vi "UDP Send and Receive (repeat on error) - I32.vi"(7 "timeout ms (100)":i32=100, 8 "error in (no error)":errorcluster, 9 "I32 Command & Param":T1, 10 "IP":string, 11 "connection ID in":refnum<k16>) -> (0 "error out":errorcluster, 2 "I32 Param out":i32, 3 "connection ID out":refnum<k16>)   [LabVIEW 2016, in "SMD-7615.lvlib" / "eSCL.lvlib"]
doc: "AC - Acceleration Rate\nSets or requests the acceleration rate used in point-to-point move commands in rev/sec/sec."
uses:
  eSCL.lvlib
  I32 Command and Param.ctl
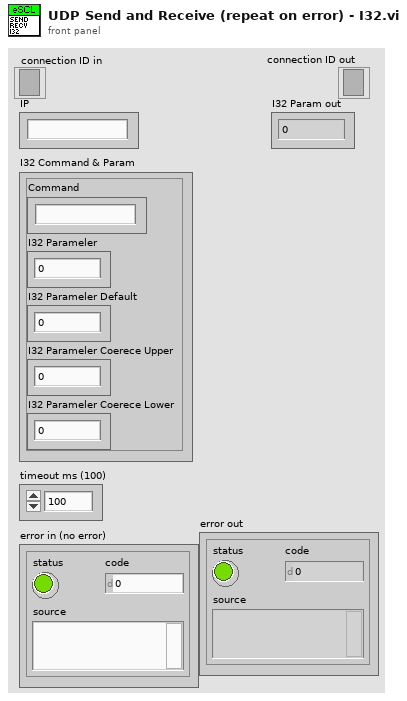
[diagram p1: front panel]
types:
  T1 = typedef "SMD-7615.lvlib/eSCL.lvlib/I32 Command and Param.ctl" = cluster{"Command":string, "I32 Parameler":i32, "I32 Parameler Default":i32, "I32 Parameler Coerece Upper":i32, "I32 Parameler Coerece Lower":i32}
  T2 = typedef "SMD-7615.lvlib/eSCL.lvlib/UDP Received Data.ctl" = cluster{"Received String":string, "eSCL Cmd":string, "Data":string}
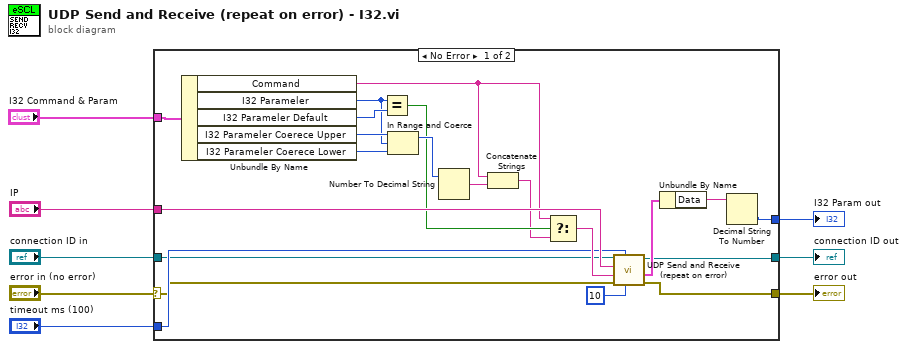
[diagram p0: block diagram]
diagram:
  n1 = case shown="No Error" "error in (no error)" {
    selector: "error in (no error)" -> [w11 w30]
    tunnel: "connection ID in" -> [w10 w31]
    tunnel: [w27 w31] -> w6
    tunnel: [w26 w30] -> w5
    tunnel: "IP" -> [w29 _]
    tunnel: "timeout ms (100)" -> [w12 _]
    tunnel: [w18 _] -> w2
    tunnel: "I32 Command & Param" -> [w25 _]
    frame No Error {
      n2 = Unbundle By Name(w25) -> ("Command"=w14:string, "I32 Parameler"=w17:i32, "I32 Parameler Default"=w22:i32, "I32 Parameler Coerece Upper"=w24:i32, "I32 Parameler Coerece Lower"=w23:i32)
      n3 = Equal?(x=w17, y=w22) -> (x = y?=w16:bool)
      n4 = In Range and Coerce(upper limit=w24, x=w17, lower limit=w23) -> (coerced(x)=w21:i32)  [unwired: 1 out]
      n5 = Number To Decimal String(number=w21) -> (decimal integer string=w20:string)  [unwired: 1 in]
      n6 = Concatenate Strings(w14, w20) -> (w15:string)
      n7 = Select(t=w14, s=w16, f=w15) -> (s? t:f=w13:string)
      n8 = call "UDP Send and Receive (repeat on error).vi"("Number of retries (3)"=u8 10, "timeout ms (100)"=w12, "error in (no error)"=w11, "Data"=w13, "IP"=w29, "connection ID in"=w10) -> ("error out"=w26:errorcluster, "Received Data"=w28:T2, "connection ID out"=w27:refnum<k16>)  [unwired: 2 in, 1 out]
      n9 = Unbundle By Name(w28) -> ("Data"=w19:string)
      n10 = Decimal String To Number(string=w19) -> (number=w18:i32)  [unwired: 2 in, 1 out]
    }
    frame Error {
    }
  }
  "connection ID out" <- w6
  "error out" <- w5
  "I32 Param out" <- w2
